vi "NoisySine.vi"() -> ()   [LabVIEW 2015]
uses:
  <vilib>/imath/engines/lvmath2/RunTimeEngine/BuiltInFunctions/randnormal/NIMS_randnormal().vi
  <vilib>/imath/engines/lvmath2/RunTimeEngine/ErrorHandling/NIMS_Error From Error Code.vi
  <vilib>/imath/engines/lvmath2/RunTimeEngine/NodeEndStatement/NIMS_NodeEndStatement_Output.vi
  <instcachedir>/0/NIMS_NodeEndStatement_Output_53EC0D466D134D7ABD903AC30B43404B.lvgen/NIMS_NodeEndStatement_Output_53EC0D466D134D7ABD903AC30B43404B_001.vi
  <vilib>/imath/engines/lvmath2/RunTimeEngine/ErrorHandling/NIMS_Finalize Error.vi
panel:
  out "XY Graph":cluster{dbl[], dbl[]}(graph)
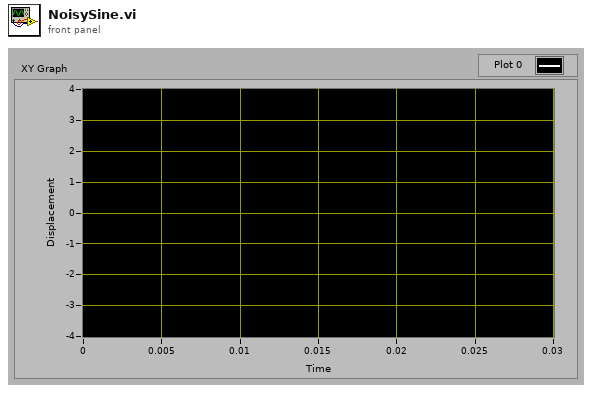
[diagram p1: front panel]
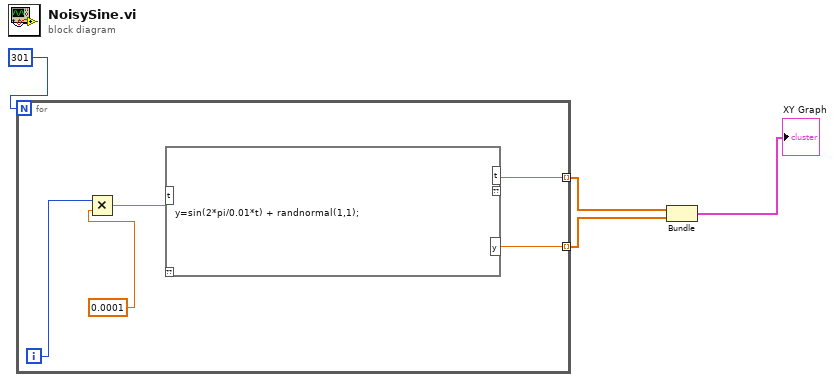
[diagram p0: block diagram]
diagram:
  n1 = for {
    N: 301 -> [_]
    tunnel: [w6] -> w3 mode=indexing
    tunnel: [w5] -> w2 mode=indexing
    i -> [w8]
    n2 = Multiply(x=w8, y=0.0001) -> (x*y=w9:dbl)
    n3 = mathscript code="y=sin(2*pi/0.01*t) + randnormal(1,1);"("t"=w9) -> ("t"=w6:dbl, "y"=w5:dbl)  [unwired: 1 in, 1 out]
  }
  n4 = Bundle(w3, w2) -> (→"XY Graph":cluster{dbl[], dbl[]})  [unwired: 1 in]
